vi "TLB Native Dynamic Events ver 0.12.vi"() -> ()   [LabVIEW 2018]
uses:
  Labview Training Phase 2/Enum Controls/States for Action Engine.ctl
  TLB Type Definitions/State Type Definitions, for 0.26g versions and later 2.ctl
  TLB Type Definitions/Intruction Type Definitions.ctl
  TLB Type Definitions/Encoder cluster.ctl
  Experimental VI's/Archived VI's/MOTOR CONTROL NO PID Type Def.ctl
  Underlying VI's/I2C Master VI/I2C MASTER Type Def.ctl
  TLB Type Definitions/PING CLUSTER.ctl
  <vilib>/Studica/Studica Toolkit/NavX/NavX.lvlib
  <vilib>/Studica/Studica Toolkit/Background/DIO Channel.ctl
  Underlying VI's/NavX VI/navX type def.ctl
  <vilib>/myRIO/Instrument Drivers/Utilities/Utilities.lvlib
  <vilib>/Studica/Studica Toolkit/Background/I2C Channel.ctl
  <vilib>/Studica/Studica Toolkit/NavX/TypeDefs/Flags/Z900_navX_Flags_CalibrationStatusTypeDef.ctl
  <vilib>/Studica/Studica Toolkit/NavX/TypeDefs/Flags/Z900_navX_Flags_OpStatusTypeDef.ctl
panel:
  out "Detect?":bool
  out "Status":T3 {"OP Status" items=["INITIALIZING", "SELFTEST_IN_PROGRESS", "ERROR", "IMU_AUTOCAL_IN_PROGRESS", "NORMAL"]; "Calibration Status" items=["IMU_CAL_STATE_MASK"=3, "IMU_CAL_STATE_INPROGRESS"=0, "IMU_CAL_STATE_ACCUMULATE"=1, "IMU_CAL_STATE_COMPLETE"=2]}
  out "NavX Readings":T4
  out "TASK ENABLE":bool
  out "Rising Edge":bool
  in  "Green LED":bool
  out "Task Selection":u8
  out "Object detected?":bool
  in  "Arduino Mode":T5=enum."Mode 0"
  out "Arduino Data":T6
  out "I2C Error":errorcluster
  out "Speed & distance":T7
  out "State Logic":T8=enum."Startup"
  out "elements":T9[](array[typedef])
  in  "STOP TASK":bool
  in  "OK Button":bool
  in  "STOP":bool
  out "error out":errorcluster
  out "Action Queue Items":i32
  out "State Logic Queue Items":i32
  out "Action Queues items":string[](array[string])=["Hardware reset", "Software reset", ""]
  out "Action State":string
  # "TLB FRAMEWORK STATUS"
  # "System Health Status Update"
  # "Test Programme written by Calvin Loke    Dated: 28 Aug 2019\nTest Programme revised by Dr Alex See   Dated 30 Aug 2019\n\nProgramme version:   TLB Native Dynamic Events ver 0.04b.vi"
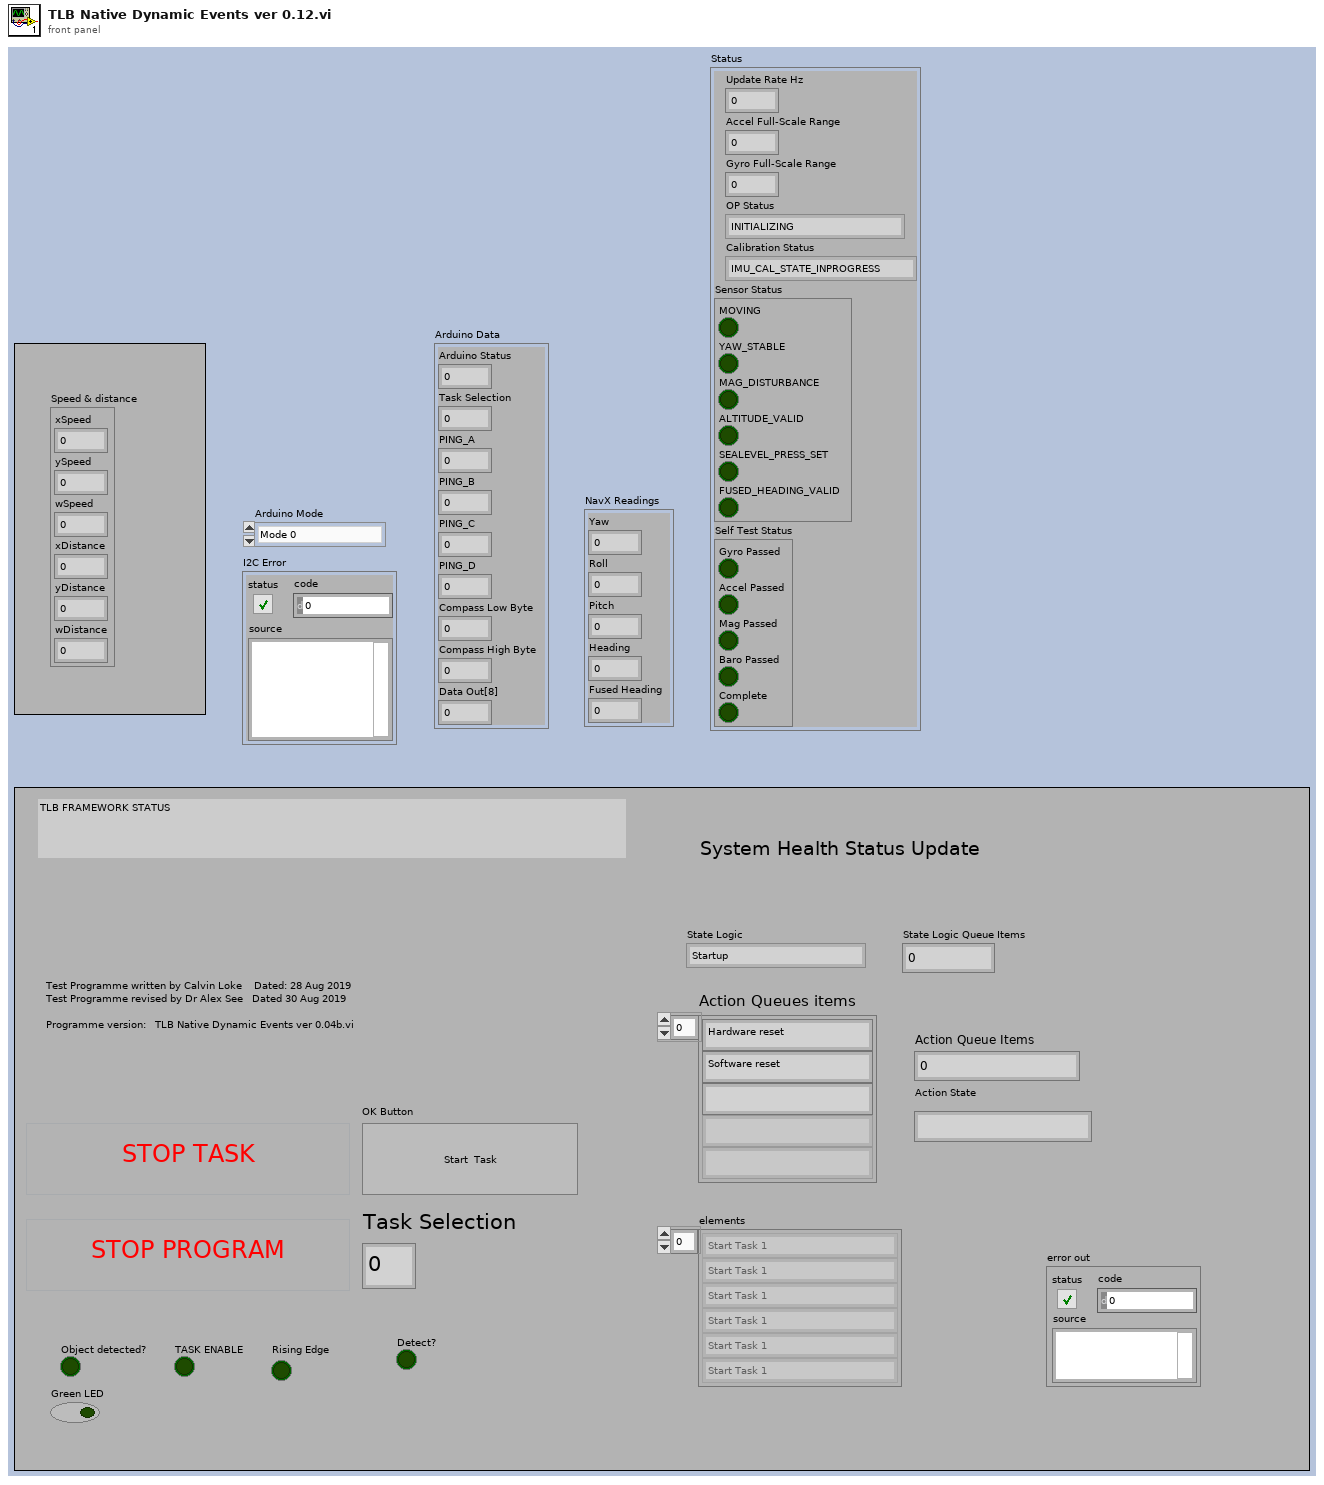
[diagram p1: front panel]
types:
  T1 = typedef "NavX.lvlib/Z900_navX_Flags_OpStatusTypeDef.ctl" = u8
  T2 = typedef "NavX.lvlib/Z900_navX_Flags_CalibrationStatusTypeDef.ctl" = u8
  T3 = cluster{"Update Rate Hz":u8, "Accel Full-Scale Range":u8, "Gyro Full-Scale Range":u16, "OP Status":T1, "Calibration Status":T2, "Sensor Status":cluster{"MOVING":bool, "YAW_STABLE":bool, "MAG_DISTURBANCE":bool, "ALTITUDE_VALID":bool, "SEALEVEL_PRESS_SET":bool, "FUSED_HEADING_VALID":bool}, "Self Test Status":cluster{"Gyro Passed":bool, "Accel Passed":bool, "Mag Passed":bool, "Baro Passed":bool, "Complete":bool}}
  T4 = cluster{"Yaw":dbl, "Roll":dbl, "Pitch":dbl, "Heading":dbl, "Fused Heading":dbl}
  T5 = typedef "I2C MASTER Type Def.ctl" = enum16{"Last State", "Mode 0", "Mode 1", "Mode 2", "Mode 3", "Mode 4", "Mode 5", "Mode 6", "Mode 7", "Mode 8", "Mode 9", "Mode 10"}
  T6 = cluster{"Arduino Status":u8, "Task Selection":u8, "PING_A":u8, "PING_B":u8, "PING_C":u8, "PING_D":u8, "Compass Low Byte":u8, "Compass High Byte":u8, "Data Out[8]":u8}
  T7 = cluster{"xSpeed":dbl, "ySpeed":dbl, "wSpeed":dbl, "xDistance":dbl, "yDistance":dbl, "wDistance":dbl}
  T8 = typedef "State Type Definitions, for 0.26g versions and later 2.ctl" = enum16{"None", "Startup", "Move to Angle", "True Stop", "Idle", "Shutdown", "Task 1A", "Task 1B", "Task 2:Raise Arm", "Task 2:Sensor Mode", "Task 2:Reverse Mode", "Task 3", "Task 4_A", "Task 4_B", "Task 4_C", "Task 4_D", "Task 5A", "Task 5B", "Task 5C", "Task 5D", "Task 5E: POSITION ARM", "Task 5F: ARM GRAB HEIGHT", "Task 5G: CLOSE CLAW", "Task 5H: RAISE ARM", "Task 6_A", "Task 6_B", "Task 7", "Task 8A: RAISE ARM", "Task 8B: MOVE TO BOX", "Task 8C: CAM BURST", "Task 8D: PROCESS IMAGE", "Task 8E: ROBOT ADJUST", "Task 8F: CAM BURST 2", "Task 8G: PROCESS IMAGE 2", "Task 8H: ARM ADJUST", "Task 8I: ARM GRAB HEIGHT", "Task 8J: CLOSE CLAW", "Task 8K: RAISE MY SWORD", "Task 9A: Raise Arm", "Task 9B: Rotate to Angle", "Task 9C: Detect Box", "Task 9D: MOVE FORWARD", "Task 9E: MOVE LEFT", "Task 9F: SCAN BOX", "Task 9G: MOVE RIGHT", "Task 9H: SCAN BOX 2", "Task 9I: ROTATE 90 CW", "Task 9J: FORWARD", "Task 9K: MOVE RIGHT", "Task 9L: SCAN BOX 3", "Task 9M: MOVE RIGHT", "Task 9N: SCAN BOX 4", "PENIS", "PENIS 2", "PENIS 3", "Task 9R: PROCESS COLOUR", "Task A1: Task 9 Open cam", "Task A2: Task 9 Move Arm", "Task A3: Task 9 Set Timer", "Task A4: Tasl 9 Capture images", "Task A5: Task 9 Close camera", "Task A6: Process Colour", "Task A7: Dispose Camera Buffer"}
  T9 = typedef "Intruction Type Definitions.ctl" = enum16{"None", "Start Task 1", "Start Task 2", "Start Task 3", "Start Task 4", "Start Task 5", "Start Task 6", "Start Task 7", "Start Task 8 - BALL", "Start Task 8 - Gel", "Start Task 8 - Pipe", "Start Task 8 - Soap", "Start Task 9", "Start Task A", "Start Task B", "Exit"}
  T10 = typedef "States for Action Engine.ctl" = enum16{"Initialize", "Write", "Read"}
  T11 = typedef "DIO Channel.ctl" = enum16{"Not Connected", "A/DIO1", "A/DIO2", "A/DIO3", "A/DIO4", "A/DIO5", "A/DIO6", "A/DIO7", "A/DIO13", "B/DIO1", "B/DIO2", "B/DIO3", "B/DIO4", "B/DIO5", "B/DIO6", "B/DIO7", "B/DIO13", "C/DIO0", "C/DIO1", "C/DIO2", "C/DIO3", "C/DIO4", "C/DIO5", "C/DIO6", "C/DIO7"}
  T12 = typedef "PING CLUSTER.ctl" = cluster{"PING_A":u8, "PING_B":u8, "PING_C":u8, "PING_D":u8}
  T13 = typedef "Encoder cluster.ctl" = cluster{"xDistance":dbl, "yDistance":dbl, "wDistance":dbl}
  T14 = typedef "I2C Channel.ctl" = enum16{"Not Connected", "A", "B"}
  T15 = typedef "navX type def.ctl" = enum16{"Get i2C reference", "Read Values", "Zero Yaw"}
  T16 = typedef "State Type Definitions.ctl" = enum16{"None", "Startup", "Move to Angle", "True Stop", "Idle", "Shutdown", "Task 1", "Task 2:Raise Arm", "Task 2:Sensor Mode", "Task 2:Reverse Mode", "Task 3", "Task 4_A", "Task 4_B", "Task 4_C", "Task 4_D", "Task 5A: ARM CAM HEIGHT", "Task 5B: MOVE TO BOX", "Task 5C: CAM BURST", "Task 5D: PROCESS IMAGE", "Task 5E: POSITION ARM", "Task 5F: ARM GRAB HEIGHT", "Task 5G: CLOSE CLAW", "Task 5H: RAISE ARM", "Task 6_A", "Task 6_B", "Task 7", "Task 8A: RAISE ARM", "Task 8B: MOVE TO BOX", "Task 8C: CAM BURST", "Task 8D: PROCESS IMAGE", "Task 8E: ROBOT ADJUST", "Task 8F: CAM BURST 2", "Task 8G: PROCESS IMAGE 2", "Task 8H: ARM ADJUST", "Task 8I: ARM GRAB HEIGHT", "Task 8J: CLOSE CLAW", "Task 8K: RAISE MY SWORD", "Task 9A: Raise Arm", "Task 9B: Rotate to Angle", "Task 9C: Detect Box", "Task 9D: MOVE FORWARD", "Task 9E: MOVE LEFT", "Task 9F: SCAN IMAGE", "Task 9G: PROCESS COLOUR", "Task 9H: MOVE RIGHT", "Task 9I: SCAN IMAGE", "Task 9J: PROCESS COLOUR", "Task 9K: ROTATE 90 CW", "Task 9L: MOVE FORWARD", "Task 9M: MOVE RIGHT", "Task 9N: SCAN IMAGE", "Task 9O: PROCESS COLOUR", "Task 9P: MOVE RIGHT", "Task 9Q: SCAN IMAGE", "Task 9R: PROCESS COLOUR"}
  T17 = typedef "State Type Definitions.ctl" = enum16{"None", "Startup", "Move to Angle", "True Stop", "Idle", "Shutdown", "Task 1", "Task 2", "Task 3", "Task 4_A", "Task 4_B", "Task 4_C", "Task 5", "Task 6", "Task 7", "Task 8", "Task 9", "Task A", "Task B"}
  T18 = typedef "MOTOR CONTROL NO PID Type Def.ctl" = enum16{"Init", "Front Back", "Left Right", "Rotate", "Stop", "Latch"}
  T19 = cluster{"DIO Channel":T11, "FPGA VI Reference Out":refnum<k20>}
  T20 = cluster{"I2C Ref Out":cluster{"I2C Channel":T14, "FPGA VI Reference Out":refnum<k20>}, "Connected":bool, "Slave Address (7-bit)":u8, "Registry":u8[]}
  T21 = cluster{"Arduino State":u8, "Rotary Switch":u8, "Ultrasonic 1":u8, "Ultrasonic 2":u8, "Ultrasonic 3":u8, "Ultrasonic 4":u8, "y Stepper Position":u8, "z Stepper Position":u8, "Data Out[8]":u8}
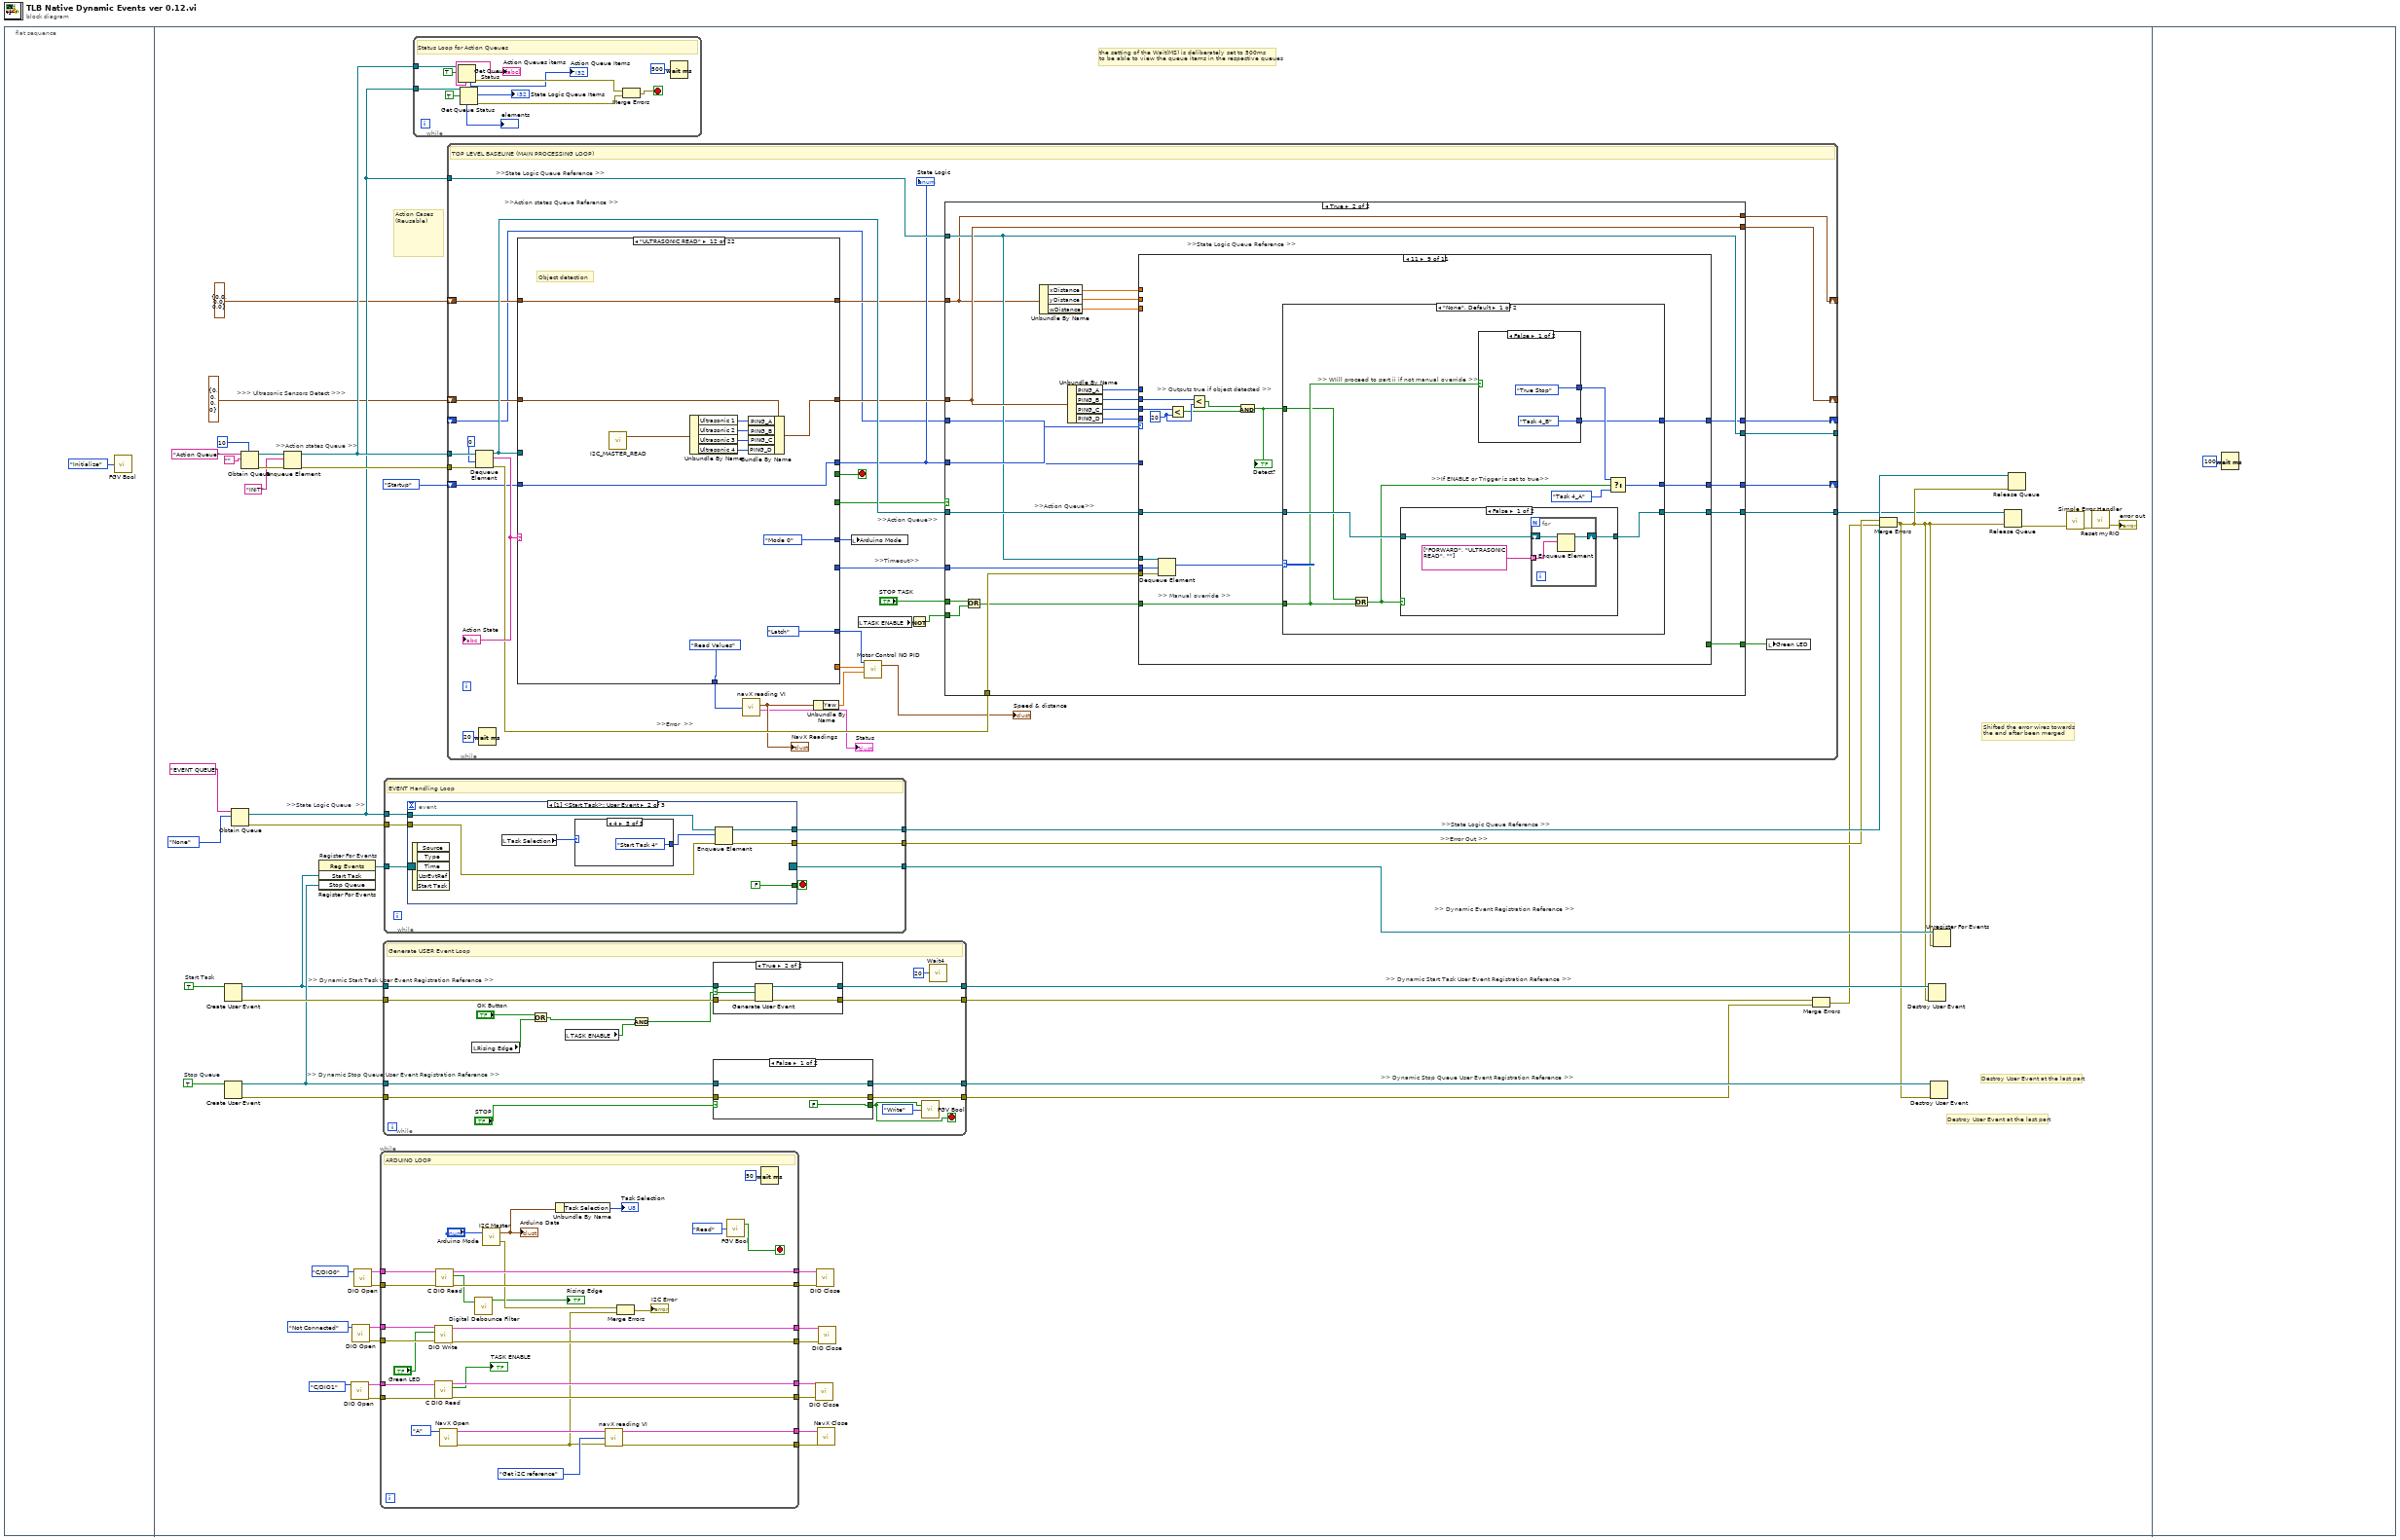
[diagram p0: block diagram]
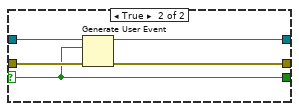
[diagram p2: hidden frame]
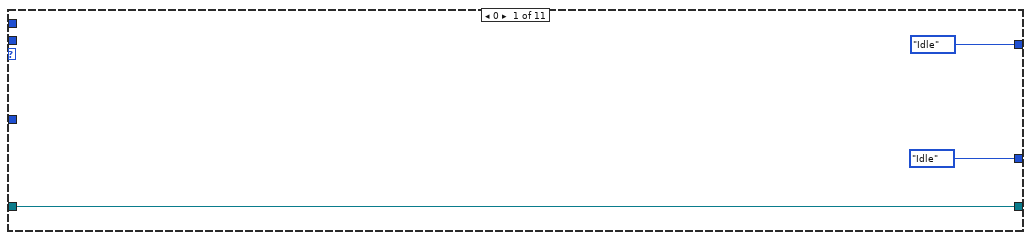
[diagram p5: hidden frame]
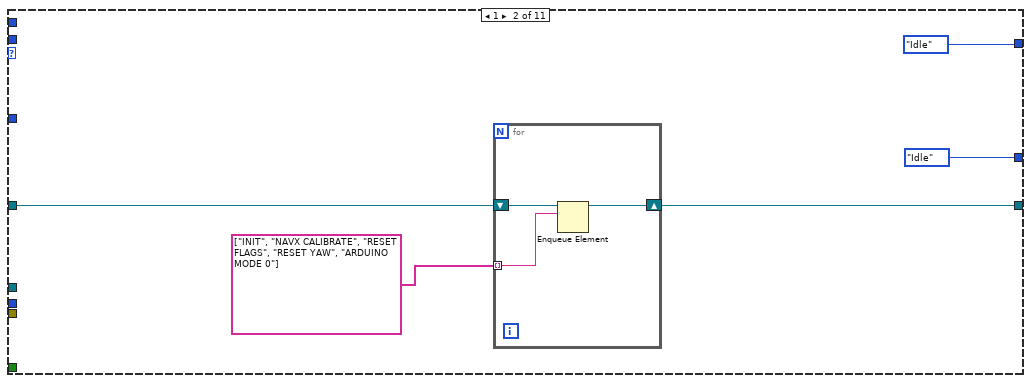
[diagram p6: hidden frame]
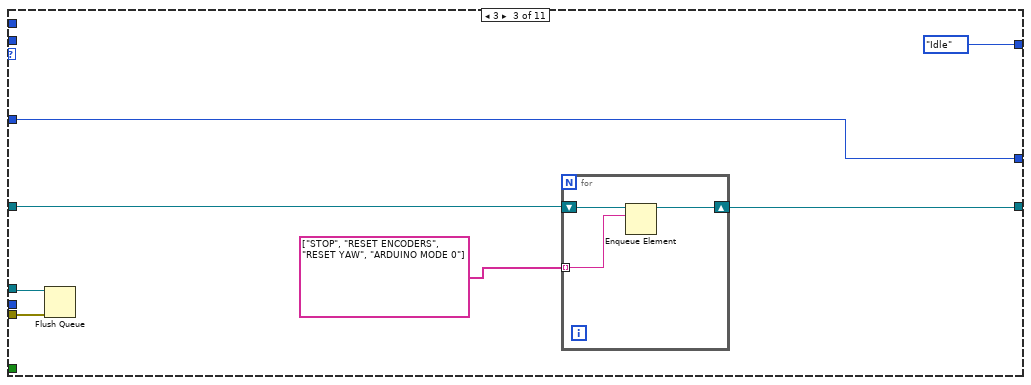
[diagram p7: hidden frame]
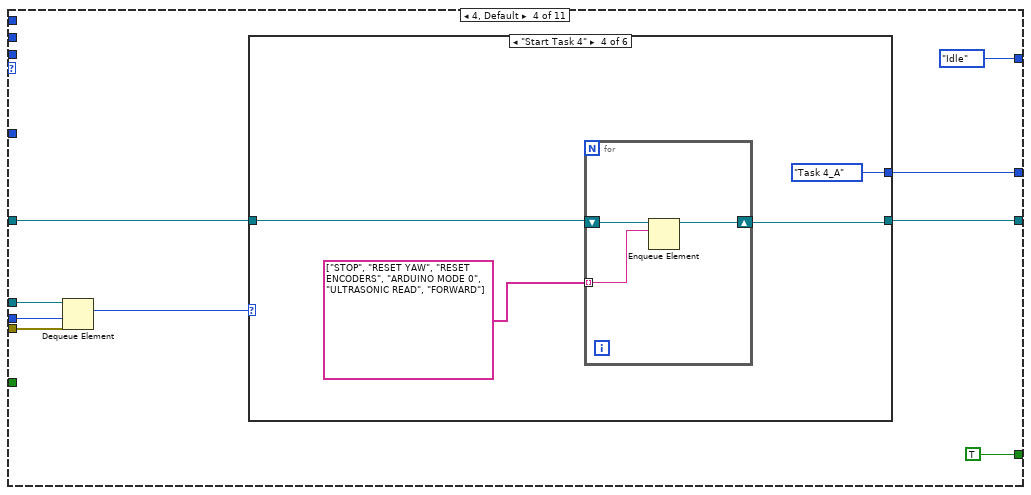
[diagram p8: hidden frame]
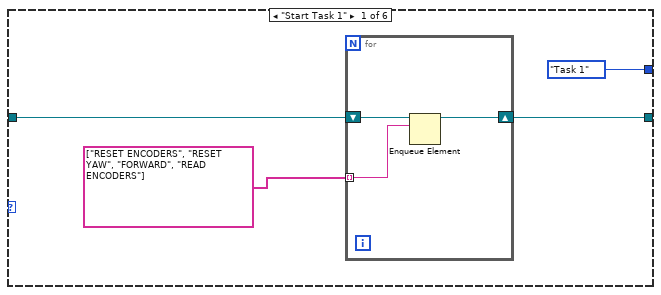
[diagram p9: hidden frame]
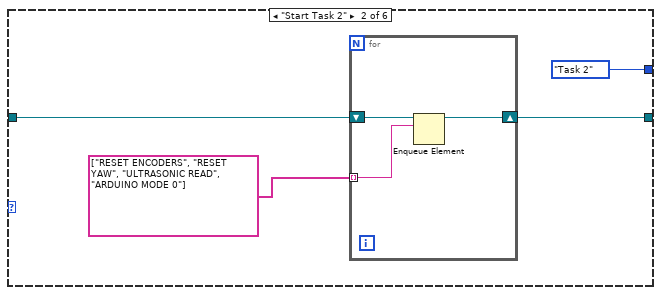
[diagram p10: hidden frame]
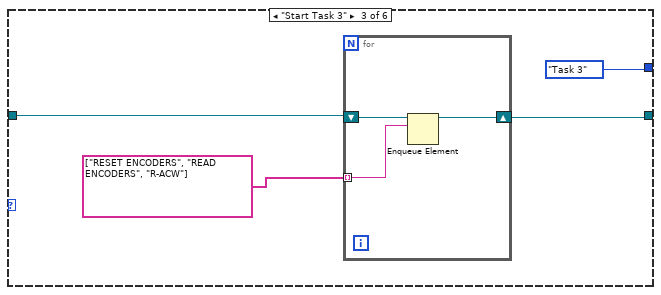
[diagram p11: hidden frame]
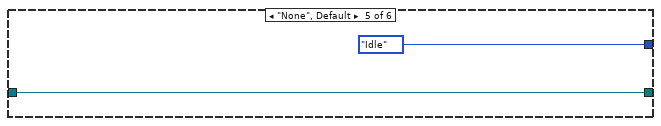
[diagram p12: hidden frame]
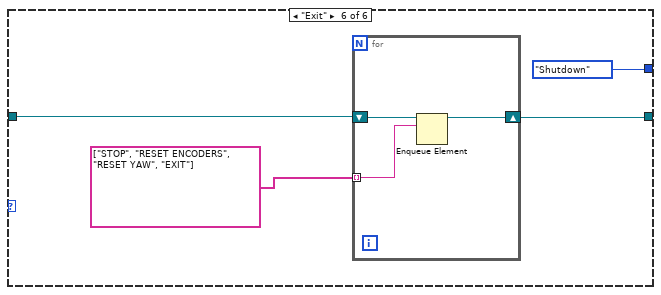
[diagram p13: hidden frame]
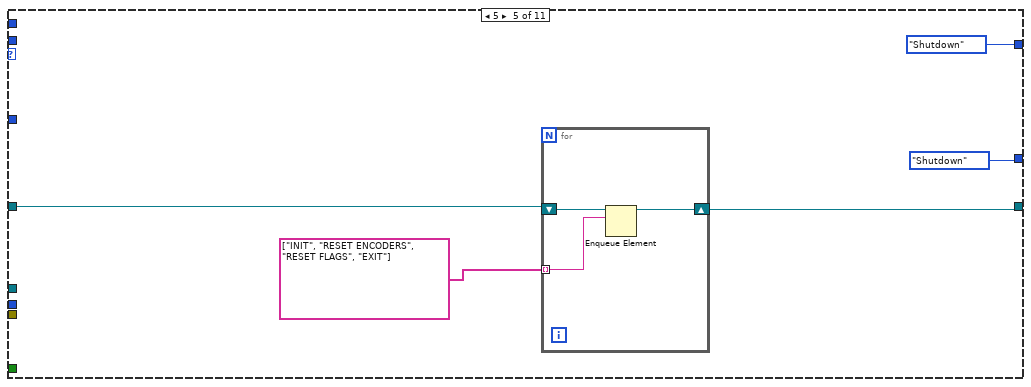
[diagram p14: hidden frame]
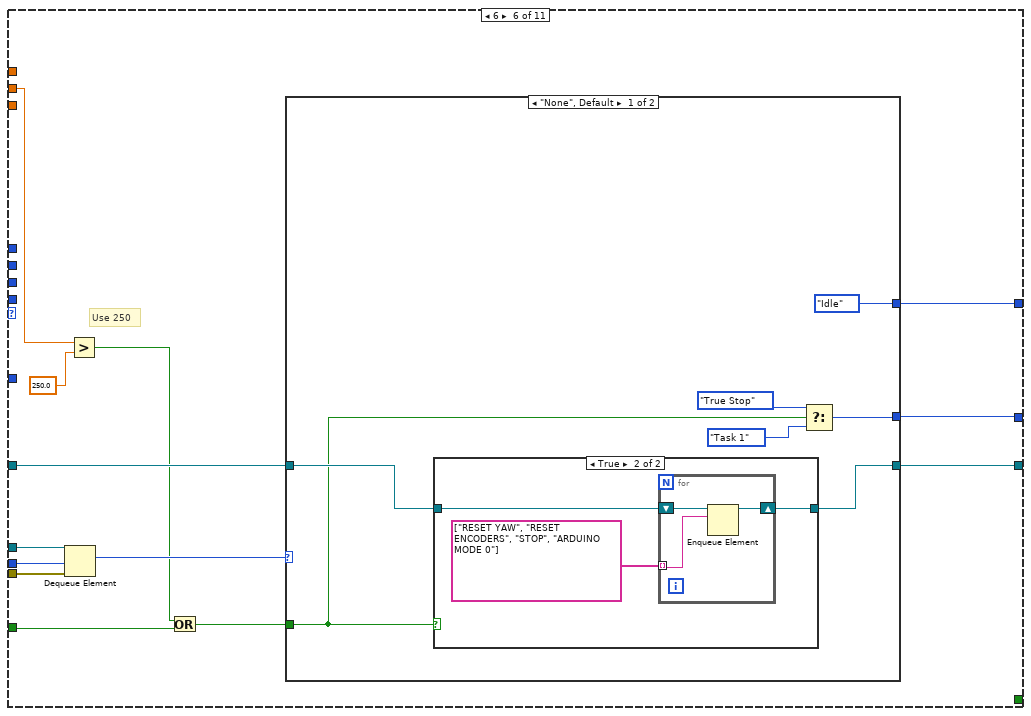
[diagram p15: hidden frame]
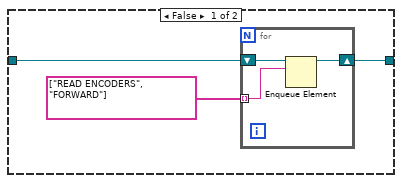
[diagram p16: hidden frame]
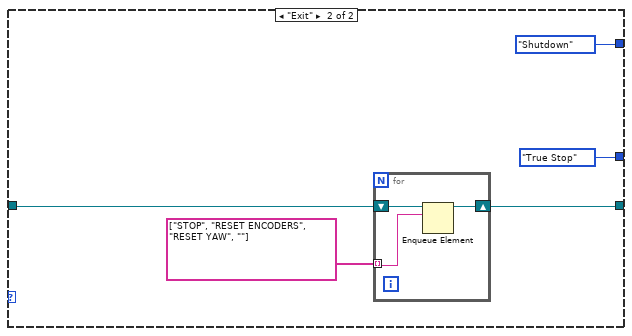
[diagram p17: hidden frame]
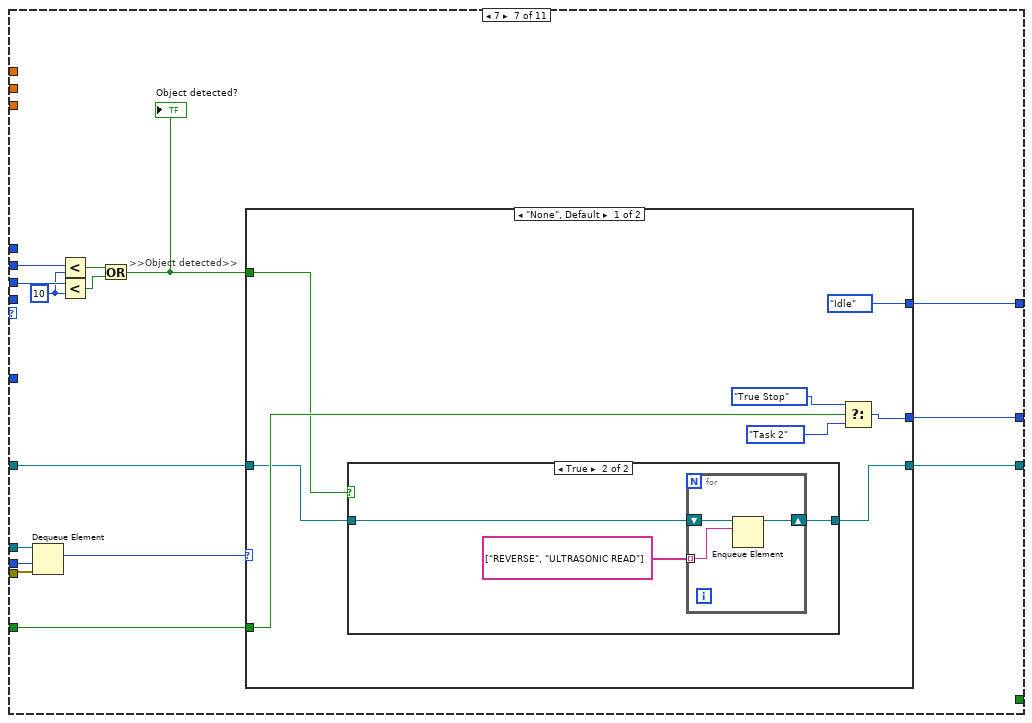
[diagram p18: hidden frame]
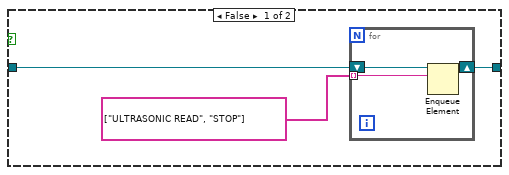
[diagram p19: hidden frame]
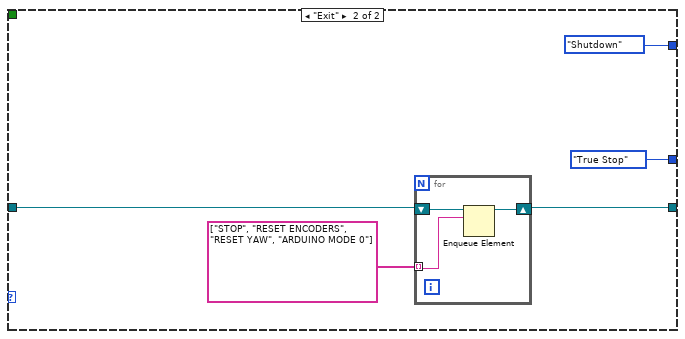
[diagram p20: hidden frame]
diagram:
  n1 = flat-sequence {
    frame #0 {
      n2 = call "FGV Bool.vi"("Init/Read/Write State"=States_for_Action_Engine."Initialize") -> ()  [unwired: 2 in, 2 out]
    }
    frame #1 {
      w53 = TRUE  # Stop Queue
      w52 = TRUE  # Start Task
      # ">>> Ultrasonic Sensors Detect >>>"
      # "the setting of the Wait(MS) is deliberately set to 500ms\nto be able to view the queue items in the respective queues"
      # "Action Cases\n(Reusable)"
      # ">>Error Out >>"
      # ">> Dynamic Stop Queue User Event Registration Reference >>"
      # ">> Dynamic Start Task User Event Registration Reference >>"
      # ">> Dynamic Stop Queue User Event Registration Reference >>"
      # ">> Dynamic Start Task User Event Registration Reference >>"
      # ">> Dynamic Event Registration Reference >>"
      # ">>Action states Queue >>"
      # ">>State Logic Queue  >>"
      # ">>State Logic Queue Reference >>"
      # "Destroy User Event at the last part"
      # "Destroy User Event at the last part"
      # "Shifted the error wires towards\nthe end after been merged"
      n3 = Create User Event(user event datatype=w52) -> (user event=w44:refnum<user-event>, error out=w49:errorcluster)  [unwired: 1 in]
      n4 = Create User Event(user event datatype=w53) -> (user event=w45:refnum<user-event>, error out=w48:errorcluster)  [unwired: 1 in]
      n5 = Obtain Queue(name (unnamed)="EVENT QUEUE", element data type=Intruction_Type_Definitions."None" ("Enum")) -> (queue out=w30:refnum<queue>, error out=w36:errorcluster)  [unwired: 3 in, 1 out]
      n6 = Obtain Queue(max queue size (-1, unlimited)=10, name (unnamed)="Action Queue", element data type="") -> (queue out=w39:refnum<queue>, error out=w35:errorcluster)  [unwired: 2 in, 1 out]
      n7 = Enqueue Element(queue=w39, element="INIT", error in (no error)=w35) -> (queue out=w31:refnum<queue>, error out=w34:errorcluster)  [unwired: 1 in, 1 out]
      n8 = register-events "Register For Events"(w44, w45) -> (reference out=w43:refnum<event-registration>)  [unwired: 2 in, 1 out]
      n9 = call <vilib>:"DIO Open.vi"("DIO Channel"=DIO_Channel."C/DIO1") -> ("error out"=w8:errorcluster, "DIO Info Out"=w9:T19)  [unwired: 9 in]
      n10 = call <vilib>:"DIO Open.vi"("DIO Channel"=DIO_Channel."Not Connected") -> ("error out"=w13:errorcluster, "DIO Info Out"=w15:T19)  [unwired: 9 in]
      n11 = call <vilib>:"DIO Open.vi"("DIO Channel"=DIO_Channel."C/DIO0") -> ("error out"=w18:errorcluster, "DIO Info Out"=w21:T19)  [unwired: 9 in]
      n12 = while {
        tunnel: w21 -> [w78]
        tunnel: [w77] -> w19
        tunnel: w18 -> [w76]
        tunnel: [w75] -> w17
        tunnel: w15 -> [w69]
        tunnel: [w68] -> w14
        tunnel: w13 -> [w67]
        tunnel: [w66] -> w12
        tunnel: [w64] -> w10
        tunnel: w9 -> [w63]
        tunnel: w8 -> [w62]
        tunnel: [w61] -> w7
        tunnel: [w58] -> w6
        tunnel: [w57] -> w5
        stop <- w82 stop-if-true
        # "ARDUINO LOOP"
        n13 = call <vilib>:"DIO Write.vi"("error in (no error)"=w67, "Input"="Green LED", "DIO Info In"=w69) -> ("error out"=w66:errorcluster, "DIO Info Out"=w68:T19)  [unwired: 7 in]
        n14 = call <vilib>:"C DIO Read.vi"("error in (no error)"=w62, "DIO Info In in"=w63) -> ("error out"=w61:errorcluster, "IN"=→"TASK ENABLE":bool, "DIO Info In out"=w64:T19)  [unwired: 7 in]
        n15 = call <vilib>:"C DIO Read.vi"("error in (no error)"=w76, "DIO Info In in"=w78) -> ("error out"=w75:errorcluster, "IN"=w72:bool, "DIO Info In out"=w77:T19)  [unwired: 7 in]
        n16 = call <vilib>:"NavX Open.vi"("I2C Channel"=I2C_Channel."A") -> ("error out"=w55:errorcluster, "NavX Info"=w59:T20)  [unwired: 9 in]
        n17 = call "Digital Debounce Filter.vi"("Boolean input"=w72) -> ("Rising Edge"=→"Rising Edge":bool)  [unwired: 1 in, 2 out]
        n18 = call "I2C Master.vi"("Arduino Mode"="Arduino Mode") -> ("I2C Error"=w74:errorcluster, "Arduino Data"=w70:T6)  [unwired: 1 in]
        "Arduino Data" <- w70
        n19 = Unbundle By Name(w70) -> ("Task Selection"=→"Task Selection":u8)
        n20 = call "navX reading VI.vi"("NavX Info In"=w59, "Mode"=navX_type_def."Get i2C reference", "error in (no error)"=w55) -> ("NavX Info Out"=w58:T20, "Error Out"=w57:errorcluster)  [unwired: 2 out]
        n21 = Merge Errors(w74, w55) -> (→"I2C Error":errorcluster)
        n22 = call "FGV Bool.vi"("Init/Read/Write State"=States_for_Action_Engine."Read") -> ("Output node"=w82:bool)  [unwired: 2 in, 1 out]
        n23 = Wait (ms)(milliseconds to wait=u32 50) -> ()  [unwired: 1 out]
      }
      n24 = while {
        tunnel: w44 -> [w112]
        tunnel: w45 -> [w111]
        tunnel: [w110] -> w51
        tunnel: [w109] -> w50
        tunnel: w49 -> [w108]
        tunnel: [w107] -> w47
        tunnel: w48 -> [w106]
        tunnel: [w105] -> w46
        stop <- w103 stop-if-true
        # "Generate USER Event Loop"
        n25 = local read "Rising Edge"() -> (w99:bool)
        n26 = Or(x="OK Button", y=w99) -> (x .or. y?=w98:bool)
        n27 = local read "TASK ENABLE"() -> (w97:bool)
        n28 = And(x=w98, y=w97) -> (x .and. y?=w96:bool)
        n29 = case shown="True" w96 {
          selector: w96 -> [_ w123]
          tunnel: w112 -> [w122 w127]
          tunnel: [w122 w126] -> w109
          tunnel: w108 -> [w121 w125]
          tunnel: [w121 w124] -> w107
          frame False {
          }
          frame True {
            n30 = Generate User Event(user event=w127, event data cluster=w123, error in=w125) -> (user event out=w126:refnum<user-event>, error out=w124:errorcluster)  [unwired: 1 in]
          }
        }
        n31 = case shown="False" "STOP" {
          selector: "STOP" -> [_ w116]
          tunnel: w111 -> [w115 w120]
          tunnel: [w115 w119] -> w110
          tunnel: w106 -> [w114 w118]
          tunnel: [w114 w117] -> w105
          tunnel: [FALSE w116] -> w103
          frame False {
          }
          frame True {
            n32 = Generate User Event(user event=w120, event data cluster=w116, error in=w118) -> (user event out=w119:refnum<user-event>, error out=w117:errorcluster)  [unwired: 1 in]
          }
        }
        n33 = call "FGV Bool.vi"("Init/Read/Write State"=States_for_Action_Engine."Write", "Input Node"=w103) -> ()  [unwired: 1 in, 2 out]
        n34 = call "Wait4"("Count(uSec)"=u32 20) -> ()  [unwired: 1 out]
      }
      n35 = while {
        tunnel: w43 -> [w685]
        tunnel: [w684] -> w42
        tunnel: w30 -> [w682]
        tunnel: [w681] -> w41
        tunnel: w36 -> [w680]
        tunnel: [w679] -> w33
        stop <- w683 stop-if-true
        # "EVENT Handling Loop"
        n36 = event shown="[1] <Start Task>: User Event" {
          selector: w685 -> [_ _ _]
          dyn-events: [_ _ _] -> w684
          timeout: _ -> [_ _ _]
          tunnel: [FALSE FALSE w709] -> w683
          tunnel: w682 -> [w690 w697 w707]
          tunnel: [w689 w696 w708] -> w681
          tunnel: w680 -> [w688 w695 w706]
          tunnel: [w687 w694 w705] -> w679
          event Timeout {
            n37 = event-data() -> ()  [unwired: 1 in, 3 out]
            n38 = Enqueue Element(queue=w690, element=Intruction_Type_Definitions."None" ("Enum"), error in (no error)=w688) -> (queue out=w689:refnum<queue>, error out=w687:errorcluster)  [unwired: 1 in, 1 out]
          }
          event User Event {
            n39 = event-data() -> ()  [unwired: 1 in, 5 out]
            n40 = local read "Task Selection"() -> (w692:u8)
            n41 = case shown="4" w692 {
              tunnel: [Intruction_Type_Definitions."None" ("Enum") Intruction_Type_Definitions."Start Task 1" ("Enum") Intruction_Type_Definitions."Start Task 2" ("Enum") Intruction_Type_Definitions."Start Task 3" ("Enum") Intruction_Type_Definitions."Start Task 4" ("Enum")] -> w693
              frame 0, Default {
              }
              frame 1 {
              }
              frame 2 {
              }
              frame 3 {
              }
              frame 4 {
              }
            }
            n42 = Enqueue Element(queue=w697, element=w693, error in (no error)=w695) -> (queue out=w696:refnum<queue>, error out=w694:errorcluster)  [unwired: 1 in, 1 out]
          }
          event User Event {
            n43 = event-data() -> ("Stop Queue"=w709:bool)  [unwired: 1 in, 4 out]
            n44 = Enqueue Element At Opposite End(queue=w707, element=Intruction_Type_Definitions."Exit" ("Enum"), error in (no error)=w706) -> (queue out=w708:refnum<queue>, error out=w705:errorcluster)  [unwired: 1 in, 1 out]
          }
        }
      }
      n45 = while {
        tunnel: w31 -> [w93]
        tunnel: w30 -> [w90]
        stop <- w87 stop-if-true
        # "Status Loop for Action Queues"
        n46 = Get Queue Status(queue=w93, return elements? (F)=TRUE) -> (error out=w89:errorcluster, # elements in queue=→"Action Queue Items":i32, elements=→"Action Queues items":string[])  [unwired: 1 in, 5 out]
        n47 = Get Queue Status(queue=w90, return elements? (F)=TRUE) -> (# pending remove=→"State Logic Queue Items":i32, error out=w88:errorcluster, elements=→"elements":T9[])  [unwired: 1 in, 5 out]
        n48 = Merge Errors(w89, w88) -> (w87:errorcluster)
        n49 = Wait (ms)(milliseconds to wait=u32 500) -> ()  [unwired: 1 out]
      }
      n50 = while {
        tunnel: w30 -> [w151]
        tunnel: w31 -> [w163]
        tunnel: w34 -> [w161]
        tunnel: [w160] -> _
        tunnel: [w159] -> w24
        shift-right: [w152] -> _
        shift-left: T12 {"PING_A"=0, "PING_B"=0, "PING_C"=0, "PING_D"=0} -> [w154]
        shift-right: [w145] -> _
        shift-left: State_Type_Definitions,_for_0.26g_versions_and_later_2."Startup" ("Enum") -> [w148]
        shift-right: [w141] -> _
        shift-left: T13 {"xDistance"=0.0, "yDistance"=0.0, "wDistance"=0.0} -> [w143]
        shift-right: [w134] -> _
        shift-left: _ -> [w133]
        stop <- w150 stop-if-true
        # ">>Error  >>"
        # ">>Action Queue>>"
        # ">>Timeout>>"
        # ">>Action states Queue Reference >>"
        # ">>State Logic Queue Reference >>"
        # "TOP LEVEL BASELINE (MAIN PROCESSING LOOP)"
        n51 = Dequeue Element(queue=w163, timeout in ms (-1)=0, error in (no error)=w161) -> (queue out=w155:refnum<queue>, element=w162:string, error out=w156:errorcluster)  [unwired: 1 out]
        "Action State" <- w162
        n52 = Wait (ms)(milliseconds to wait=u32 20) -> ()  [unwired: 1 out]
        n53 = case shown="\"ULTRASONIC READ\"" w162 {
          tunnel: [_ _ _ _ _ _ _ _ _ _ _ _ _ _ _ _ 0 w652 _ _ _ _] -> w158
          tunnel: w155 -> [_ _ _ _ _ _ _ _ _ _ _ _ _ _ _ _ _ _ _ _ _ _]
          tunnel: w154 -> [w540 w545 w552 w558 w564 w569 w576 w583 w589 w592 w604 w615 w619 w629 w633 w637 w645 w653 w658 w663 w670 w678]
          tunnel: [w540 w545 w552 w558 w564 w569 w576 w583 w589 w592 w604 w616 w619 w630 w633 w637 w645 w653 w658 w663 w669 w678] -> w153
          tunnel: [TRUE TRUE _ _ _ _ _ _ _ _ _ _ _ _ _ _ _ _ _ _ _ _] -> w150
          tunnel: w148 -> [w538 w543 w551 w557 w563 w568 w575 w582 w588 w591 w603 w614 w618 w628 w632 w636 w642 w650 w657 w662 w668 w677]
          tunnel: [_ _ _ _ _ _ _ _ _ _ _ _ _ _ _ _ _ TRUE _ _ _ _] -> w147
          tunnel: [w538 w543 w551 w557 w563 w568 w575 w582 w588 w591 w603 w614 w618 w628 w632 w636 w642 w650 w657 w662 w668 w677] -> w146
          tunnel: w143 -> [w537 w542 w550 w556 w562 w567 w574 w581 w587 w593 w602 w613 w620 w627 w634 w638 w641 w649 w659 w664 w667 w676]
          tunnel: [w537 w542 w550 w556 w562 w567 w574 w581 w587 w593 w601 w613 w620 w626 w634 w638 w641 w649 w659 w664 w667 w676] -> w142
          tunnel: [_ _ 0.4 ("Speed") -0.3 ("Speed") 0.19999999999999998 ("Speed") -0.2 ("Speed") _ 0.3 ("Speed") -0.5 ("Speed") _ _ _ _ 0.0 ("Speed") _ _ _ _ _ _ _ _] -> w140
          tunnel: [_ _ MOTOR_CONTROL_NO_PID_Type_Def."Front Back" ("Direction") _ MOTOR_CONTROL_NO_PID_Type_Def."Rotate" ("Direction") _ MOTOR_CONTROL_NO_PID_Type_Def."Stop" ("Direction") MOTOR_CONTROL_NO_PID_Type_Def."Left Right" ("Direction") MOTOR_CONTROL_NO_PID_Type_Def."Front Back" ("Direction") _ MOTOR_CONTROL_NO_PID_Type_Def."Latch" ("Direction") MOTOR_CONTROL_NO_PID_Type_Def."Latch" ("Direction") _ _ _ _ _ MOTOR_CONTROL_NO_PID_Type_Def."Latch" ("Direction") _ MOTOR_CONTROL_NO_PID_Type_Def."Init" ("Direction") _ MOTOR_CONTROL_NO_PID_Type_Def."Init" ("Direction")] -> w138
          tunnel: [I2C_MASTER_Type_Def."Last State" ("Arduino Mode") I2C_MASTER_Type_Def."Last State" ("Arduino Mode") I2C_MASTER_Type_Def."Last State" ("Arduino Mode") I2C_MASTER_Type_Def."Last State" ("Arduino Mode") I2C_MASTER_Type_Def."Last State" ("Arduino Mode") I2C_MASTER_Type_Def."Last State" ("Arduino Mode") I2C_MASTER_Type_Def."Last State" ("Arduino Mode") I2C_MASTER_Type_Def."Last State" ("Arduino Mode") I2C_MASTER_Type_Def."Last State" ("Arduino Mode") I2C_MASTER_Type_Def."Last State" ("Arduino Mode") I2C_MASTER_Type_Def."Last State" ("Arduino Mode") I2C_MASTER_Type_Def."Mode 0" ("Arduino Mode") I2C_MASTER_Type_Def."Last State" ("Arduino Mode") I2C_MASTER_Type_Def."Last State" ("Arduino Mode") I2C_MASTER_Type_Def."Mode 0" ("Arduino Mode") I2C_MASTER_Type_Def."Mode 1" ("Arduino Mode") I2C_MASTER_Type_Def."Last State" ("Arduino Mode") I2C_MASTER_Type_Def."Last State" ("Arduino Mode") I2C_MASTER_Type_Def."Last State" ("Arduino Mode") I2C_MASTER_Type_Def."Last State" ("Arduino Mode") I2C_MASTER_Type_Def."Last State" ("Arduino Mode") I2C_MASTER_Type_Def."Last State" ("Arduino Mode")] -> w137
          tunnel: [_ _ navX_type_def."Read Values" ("Mode") navX_type_def."Read Values" ("Mode") _ _ navX_type_def."Read Values" ("Mode") navX_type_def."Read Values" ("Mode") _ _ navX_type_def."Read Values" ("Mode") navX_type_def."Read Values" ("Mode") _ navX_type_def."Zero Yaw" ("Mode") _ _ navX_type_def."Zero Yaw" ("Mode") navX_type_def."Read Values" ("Mode") _ _ _ navX_type_def."Zero Yaw" ("Mode")] -> w131
          frame "Exit" {
          }
          frame "----Movement States----" {
          }
          frame "FORWARD" {
          }
          frame "LEFT" {
          }
          frame "R-ACW" {
          }
          frame "R-CW" {
          }
          frame "STOP" {
            n54 = Wait (ms)(milliseconds to wait=u32 200) -> ()  [unwired: 1 out]
          }
          frame "RIGHT" {
          }
          frame "REVERSE" {
          }
          frame "----SENSOR READING---- " {
          }
          frame "READ ENCODERS" {
            # ">>> Current encoder distance >>>"
            # ">>> Ultrasonic Sensors Detect >>>"
            n55 = local read "Speed & distance"() -> (w600:T7)
            n56 = Unbundle By Name(w600) -> ("xDistance"=w599:dbl, "yDistance"=w598:dbl, "wDistance"=w597:dbl)
            n57 = Bundle By Name(cluster=w602, "xDistance"=w599, "yDistance"=w598, "wDistance"=w597) -> (w601:T13)
          }
          frame "ULTRASONIC READ" {
            # "Object detection"
            n58 = call "I2C_MASTER_READ.vi"() -> ("Arduino Data"=w609:T21)  [unwired: 1 in, 1 out]
            n59 = Unbundle By Name(w609) -> ("Ultrasonic 1"=w608:u8, "Ultrasonic 2"=w607:u8, "Ultrasonic 3"=w606:u8, "Ultrasonic 4"=w605:u8)
            n60 = Bundle By Name(cluster=w615, "PING_A"=w608, "PING_B"=w607, "PING_C"=w606, "PING_D"=w605) -> (w616:T12)
          }
          frame "----SYSTEM MODES----" {
          }
          frame "INIT" {
            w623 = 0
            w625 = 0.0
            # ">>State Logic  >>"
            n61 = Bundle By Name(cluster=w629, "PING_A"=w623, "PING_B"=w623, "PING_C"=w623, "PING_D"=w623) -> (w630:T12)
            n62 = Bundle By Name(cluster=w627, "xDistance"=w625, "yDistance"=w625, "wDistance"=w625) -> (w626:T13)
          }
          frame "ARDUINO MODE 0" {
          }
          frame "ARDUINO MODE 1" {
          }
          frame "NAVX CALIBRATE" {
            # "Adds a 15 second delay to the startup process \nfor the NavX to calibrate"
            n63 = Wait (ms)(milliseconds to wait=u32 5000) -> ()  [unwired: 1 out]
          }
          frame "NO ACTION", Default {
            n64 = case shown="4" w650 {
              tunnel: [0 100] -> w652
              frame 1, Default {
              }
              frame 4 {
              }
            }
          }
          frame "----RESET CASES----" {
          }
          frame "RESET ENCODERS" {
          }
          frame "RESET FLAGS" {
            w666 = 0
            # "Resets any software variables\nand/or non-critical states"
            n65 = Wait (ms)(milliseconds to wait=u32 20) -> ()  [unwired: 1 out]
            n66 = Bundle By Name(cluster=w670, "PING_A"=w666, "PING_B"=w666, "PING_C"=w666, "PING_D"=w666) -> (w669:T12)
          }
          frame "RESET YAW" {
            n67 = Wait (ms)(milliseconds to wait=u32 100) -> ()  [unwired: 1 out]
          }
        }
        "State Logic" <- w146
        n68 = call "navX reading VI.vi"("Mode"=w131) -> ("NavX Readings"=w132:T4, "Status"=→"Status":T3)  [unwired: 2 in, 2 out]
        "NavX Readings" <- w132
        n69 = Unbundle By Name(w132) -> ("Yaw"=w130:dbl)
        n70 = local write "Arduino Mode"(w137) -> ()
        n71 = local read "TASK ENABLE"() -> (w136:bool)
        n72 = call "Motor Control NO PID.vi"("Yaw"=w130, "Speed"=w140, "Direction"=w138) -> ("Speed & distance"=→"Speed & distance":T7)  [unwired: 1 in, 1 out]
        n73 = Not(x=w136) -> (.not. x?=w135:bool)
        n74 = case shown="True" w147 {
          tunnel: w151 -> [w169 w186]
          tunnel: w155 -> [w165 w188]
          tunnel: [w169 w186] -> w160
          tunnel: [w165 w189] -> w159
          tunnel: w156 -> [_ w184]
          tunnel: w158 -> [_ w185]
          tunnel: w153 -> [w168 w191]
          tunnel: [w168 w191] -> w152
          tunnel: "STOP TASK" -> [_ w174]
          tunnel: w146 -> [w167 w190]
          tunnel: [w167 w187] -> w145
          tunnel: w142 -> [w166 w180]
          tunnel: [w166 w180] -> w141
          tunnel: w135 -> [_ w175]
          tunnel: [w164 w172] -> w134
          tunnel: w133 -> [w164 w171]
          tunnel: [_ w170] -> w128
          frame False {
          }
          frame True {
            # ">>Action Queue>>"
            # ">>State Logic Queue Reference >>"
            n75 = Or(x=w174, y=w175) -> (x .or. y?=w173:bool)
            n76 = Unbundle By Name(w180) -> ("xDistance"=w177:dbl, "yDistance"=w178:dbl, "wDistance"=w179:dbl)
            n77 = Unbundle By Name(w191) -> ("PING_A"=w183:u8, "PING_B"=w182:u8, "PING_C"=w181:u8, "PING_D"=w176:u8)
            n78 = case shown="11" w190 {
              tunnel: [w193 w196 w207 w215 w260 w272 w308 w354 w398 w455 w492] -> w189
              tunnel: w188 -> [w193 w199 w208 w218 w262 w273 w309 w355 w404 w448 w496]
              tunnel: [State_Type_Definitions,_for_0.26g_versions_and_later_2."Idle" ("Enum") State_Type_Definitions,_for_0.26g_versions_and_later_2."Idle" ("Enum") w203 w217 State_Type_Definitions,_for_0.26g_versions_and_later_2."Shutdown" ("Enum") w274 w311 w353 w399 w454 w493] -> w187
              tunnel: w186 -> [_ _ w206 w221 _ w279 w321 w362 w403 w452 w497]
              tunnel: w185 -> [_ _ _ w220 _ w278 w320 w361 w402 w451 w489]
              tunnel: w184 -> [_ _ w205 w216 _ w277 w319 w360 w401 w450 w488]
              tunnel: w173 -> [_ _ _ _ _ w271 w310 w357 w397 w453 w494]
              tunnel: w183 -> [_ _ _ _ _ _ _ _ _ _ _]
              tunnel: w182 -> [_ _ _ _ _ _ w317 _ w395 w443 w499]
              tunnel: w181 -> [_ _ _ _ _ _ w316 _ w396 w444 w498]
              tunnel: w179 -> [_ _ _ _ _ _ _ w359 _ _ _]
              tunnel: w178 -> [_ _ _ _ _ w270 _ _ _ _ _]
              tunnel: w177 -> [_ _ _ _ _ _ _ _ _ w439 _]
              tunnel: w176 -> [_ _ _ _ _ _ _ _ _ _ _]
              tunnel: [State_Type_Definitions,_for_0.26g_versions_and_later_2."Idle" ("Enum") State_Type_Definitions,_for_0.26g_versions_and_later_2."Idle" ("Enum") State_Type_Definitions,_for_0.26g_versions_and_later_2."Idle" ("Enum") State_Type_Definitions,_for_0.26g_versions_and_later_2."Idle" ("Enum") State_Type_Definitions,_for_0.26g_versions_and_later_2."Shutdown" ("Enum") w267 w307 w350 w390 w438 w491] -> w172
              tunnel: w171 -> [_ _ w203 _ _ _ _ _ _ _ _]
              tunnel: [_ _ _ TRUE ("Green LED") _ _ _ _ _ _ _] -> w170
              frame 0 {
              }
              frame 1 {
                n79 = for {
                  shift-right: [w202] -> w196
                  shift-left: w199 -> [w201]
                  tunnel: string[] ["INIT", "NAVX CALIBRATE", "RESET FLAGS", "RESET YAW", "ARDUINO MODE 0"] -> [w200] mode=indexing
                  n80 = Enqueue Element(queue=w201, element=w200) -> (queue out=w202:refnum<queue>)  [unwired: 2 in, 2 out]
                }
              }
              frame 3 {
                n81 = Flush Queue(queue=w206, error in (no error)=w205) -> ()  [unwired: 3 out]
                n82 = for {
                  shift-right: [w212] -> w207
                  shift-left: w208 -> [w211]
                  tunnel: string[] ["STOP", "RESET ENCODERS", "RESET YAW", "ARDUINO MODE 0"] -> [w210] mode=indexing
                  n83 = Enqueue Element(queue=w211, element=w210) -> (queue out=w212:refnum<queue>)  [unwired: 2 in, 2 out]
                }
              }
              frame 4, Default {
                n84 = Dequeue Element(queue=w221, timeout in ms (-1)=w220, error in (no error)=w216) -> (element=w219:T9)  [unwired: 3 out]
                n85 = case shown="\"Start Task 4\"" w219 {
                  tunnel: [w223 w230 w237 w244 w251 w253] -> w215
                  tunnel: w218 -> [w224 w231 w238 w245 w251 w254]
                  tunnel: [State_Type_Definitions."Task 1" ("Enum") State_Type_Definitions."Task 2" ("Enum") State_Type_Definitions,_for_0.26g_versions_and_later_2."Task 3" ("Enum") State_Type_Definitions,_for_0.26g_versions_and_later_2."Task 4_A" ("Enum") State_Type_Definitions,_for_0.26g_versions_and_later_2."Idle" ("Enum") State_Type_Definitions,_for_0.26g_versions_and_later_2."Shutdown" ("Enum")] -> w217
                  frame "Start Task 1" {
                    n86 = for {
                      shift-right: [w228] -> w223
                      shift-left: w224 -> [w227]
                      tunnel: string[] ["RESET ENCODERS", "RESET YAW", "FORWARD", "READ ENCODERS"] -> [w226] mode=indexing
                      n87 = Enqueue Element(queue=w227, element=w226) -> (queue out=w228:refnum<queue>)  [unwired: 2 in, 2 out]
                    }
                  }
                  frame "Start Task 2" {
                    n88 = for {
                      shift-right: [w235] -> w230
                      shift-left: w231 -> [w234]
                      tunnel: string[] ["RESET ENCODERS", "RESET YAW", "ULTRASONIC READ", "ARDUINO MODE 0"] -> [w233] mode=indexing
                      n89 = Enqueue Element(queue=w234, element=w233) -> (queue out=w235:refnum<queue>)  [unwired: 2 in, 2 out]
                    }
                  }
                  frame "Start Task 3" {
                    n90 = for {
                      shift-right: [w242] -> w237
                      shift-left: w238 -> [w241]
                      tunnel: string[] ["RESET ENCODERS", "READ ENCODERS", "R-ACW"] -> [w240] mode=indexing
                      n91 = Enqueue Element(queue=w241, element=w240) -> (queue out=w242:refnum<queue>)  [unwired: 2 in, 2 out]
                    }
                  }
                  frame "Start Task 4" {
                    n92 = for {
                      shift-right: [w249] -> w244
                      shift-left: w245 -> [w248]
                      tunnel: string[] ["STOP", "RESET YAW", "RESET ENCODERS", "ARDUINO MODE 0", "ULTRASONIC READ", "FORWARD"] -> [w247] mode=indexing
                      n93 = Enqueue Element(queue=w248, element=w247) -> (queue out=w249:refnum<queue>)  [unwired: 2 in, 2 out]
                    }
                  }
                  frame "None", Default {
                  }
                  frame "Exit" {
                    n94 = for {
                      shift-right: [w258] -> w253
                      shift-left: w254 -> [w257]
                      tunnel: string[] ["STOP", "RESET ENCODERS", "RESET YAW", "EXIT"] -> [w256] mode=indexing
                      n95 = Enqueue Element(queue=w257, element=w256) -> (queue out=w258:refnum<queue>)  [unwired: 2 in, 2 out]
                    }
                  }
                }
              }
              frame 5 {
                n96 = for {
                  shift-right: [w266] -> w260
                  shift-left: w262 -> [w265]
                  tunnel: string[] ["INIT", "RESET ENCODERS", "RESET FLAGS", "EXIT"] -> [w264] mode=indexing
                  n97 = Enqueue Element(queue=w265, element=w264) -> (queue out=w266:refnum<queue>)  [unwired: 2 in, 2 out]
                }
              }
              frame 6 {
                # "Use 250"
                n98 = Dequeue Element(queue=w279, timeout in ms (-1)=w278, error in (no error)=w277) -> (element=w276:T9)  [unwired: 3 out]
                n99 = Greater?(x=w270, y=250.0) -> (0:w268:bool)
                n100 = Or(x=w268, y=w271) -> (x .or. y?=w275:bool)
                n101 = case shown="\"None\", Default" w276 {
                  tunnel: w275 -> [w282 _]
                  tunnel: [w286 State_Type_Definitions,_for_0.26g_versions_and_later_2."True Stop" ("Enum")] -> w274
                  tunnel: w273 -> [w283 w301]
                  tunnel: [w281 w300] -> w272
                  tunnel: [State_Type_Definitions,_for_0.26g_versions_and_later_2."Idle" ("Enum") State_Type_Definitions,_for_0.26g_versions_and_later_2."Shutdown" ("Enum")] -> w267
                  frame "None", Default {
                    n102 = case shown="True" w282 {
                      tunnel: w283 -> [w289 w295]
                      tunnel: [w288 w293] -> w281
                      frame False {
                        n103 = for {
                          shift-right: [w291] -> w288
                          shift-left: w289 -> [w292]
                          tunnel: string[] ["READ ENCODERS", "FORWARD"] ("element") -> [w290] mode=indexing
                          n104 = Enqueue Element(queue=w292, element=w290) -> (queue out=w291:refnum<queue>)  [unwired: 2 in, 2 out]
                        }
                      }
                      frame True {
                        n105 = for {
                          shift-right: [w297] -> w293
                          shift-left: w295 -> [w298]
                          tunnel: string[] ["RESET YAW", "RESET ENCODERS", "STOP", "ARDUINO MODE 0"] -> [w296] mode=indexing
                          n106 = Enqueue Element(queue=w298, element=w296) -> (queue out=w297:refnum<queue>)  [unwired: 2 in, 2 out]
                        }
                      }
                    }
                    n107 = Select(t=State_Type_Definitions,_for_0.26g_versions_and_later_2."True Stop" ("Enum"), s=w282, f=State_Type_Definitions."Task 1" ("Enum")) -> (s? t:f=w286:u16)
                  }
                  frame "Exit" {
                    n108 = for {
                      shift-right: [w305] -> w300
                      shift-left: w301 -> [w306]
                      tunnel: string[] ["STOP", "RESET ENCODERS", "RESET YAW", ""] -> [w304] mode=indexing
                      n109 = Enqueue Element(queue=w306, element=w304) -> (queue out=w305:refnum<queue>)  [unwired: 2 in, 2 out]
                    }
                  }
                }
              }
              frame 7 {
                w315 = u16 10 ("y")
                # ">>Object detected>>"
                n110 = Dequeue Element(queue=w321, timeout in ms (-1)=w320, error in (no error)=w319) -> (element=w318:T9)  [unwired: 3 out]
                n111 = Less?(x=w317, y=w315) -> (x < y?=w314:bool)
                n112 = Less?(x=w316, y=w315) -> (x < y?=w313:bool)
                n113 = Or(x=w314, y=w313) -> (x .or. y?=w312:bool)
                "Object detected?" <- w312
                n114 = case shown="\"None\", Default" w318 {
                  tunnel: w312 -> [w325 _]
                  tunnel: [w327 State_Type_Definitions,_for_0.26g_versions_and_later_2."True Stop" ("Enum")] -> w311
                  tunnel: w310 -> [w326 _]
                  tunnel: w309 -> [w324 w344]
                  tunnel: [w323 w345] -> w308
                  tunnel: [State_Type_Definitions,_for_0.26g_versions_and_later_2."Idle" ("Enum") State_Type_Definitions,_for_0.26g_versions_and_later_2."Shutdown" ("Enum")] -> w307
                  frame "None", Default {
                    n115 = case shown="True" w325 {
                      tunnel: w324 -> [w331 w338]
                      tunnel: [w332 w337] -> w323
                      frame False {
                        n116 = for {
                          tunnel: string[] ["ULTRASONIC READ", "STOP"] ("element") -> [w333] mode=indexing
                          shift-right: [w335] -> w332
                          shift-left: w331 -> [w334]
                          n117 = Enqueue Element(queue=w334, element=w333) -> (queue out=w335:refnum<queue>)  [unwired: 2 in, 2 out]
                        }
                      }
                      frame True {
                        n118 = for {
                          shift-right: [w340] -> w337
                          shift-left: w338 -> [w341]
                          tunnel: string[] ["REVERSE", "ULTRASONIC READ"] -> [w339] mode=indexing
                          n119 = Enqueue Element(queue=w341, element=w339) -> (queue out=w340:refnum<queue>)  [unwired: 2 in, 2 out]
                        }
                      }
                    }
                    n120 = Select(t=State_Type_Definitions,_for_0.26g_versions_and_later_2."True Stop" ("Enum"), s=w326, f=State_Type_Definitions."Task 2" ("Enum")) -> (s? t:f=w327:u16)
                  }
                  frame "Exit" {
                    n121 = for {
                      shift-right: [w348] -> w345
                      shift-left: w344 -> [w349]
                      tunnel: string[] ["STOP", "RESET ENCODERS", "RESET YAW", "ARDUINO MODE 0"] -> [w347] mode=indexing
                      n122 = Enqueue Element(queue=w349, element=w347) -> (queue out=w348:refnum<queue>)  [unwired: 2 in, 2 out]
                    }
                  }
                }
              }
              frame 10 {
                n123 = Dequeue Element(queue=w362, timeout in ms (-1)=w361, error in (no error)=w360) -> (element=w351:T9)  [unwired: 3 out]
                n124 = Greater?(x=w359, y=150.0) -> (0:w356:bool)
                n125 = Or(x=w356, y=w357) -> (x .or. y?=w352:bool)
                n126 = case shown="\"Exit\"" w351 {
                  tunnel: w352 -> [w365 _]
                  tunnel: [w369 State_Type_Definitions,_for_0.26g_versions_and_later_2."True Stop" ("Enum")] -> w353
                  tunnel: w355 -> [w366 w385]
                  tunnel: [w364 w384] -> w354
                  tunnel: [State_Type_Definitions,_for_0.26g_versions_and_later_2."Idle" ("Enum") State_Type_Definitions,_for_0.26g_versions_and_later_2."Shutdown" ("Enum")] -> w350
                  frame "None", Default {
                    n127 = case shown="False" w365 {
                      tunnel: w366 -> [w372 w378]
                      tunnel: [w371 w376] -> w364
                      frame False {
                        n128 = for {
                          shift-right: [w374] -> w371
                          shift-left: w372 -> [w375]
                          tunnel: string[] ["READ ENCODERS", "R-ACW"] ("element") -> [w373] mode=indexing
                          n129 = Enqueue Element(queue=w375, element=w373) -> (queue out=w374:refnum<queue>)  [unwired: 2 in, 2 out]
                        }
                      }
                      frame True {
                        n130 = for {
                          shift-right: [w380] -> w376
                          shift-left: w378 -> [w381]
                          tunnel: string[] ["RESET YAW", "RESET ENCODERS", "STOP", "ARDUINO MODE 0"] -> [w379] mode=indexing
                          n131 = Enqueue Element(queue=w381, element=w379) -> (queue out=w380:refnum<queue>)  [unwired: 2 in, 2 out]
                        }
                      }
                    }
                    n132 = Select(t=State_Type_Definitions,_for_0.26g_versions_and_later_2."True Stop" ("Enum"), s=w365, f=State_Type_Definitions,_for_0.26g_versions_and_later_2."Task 3" ("Enum")) -> (s? t:f=w369:T8)
                  }
                  frame "Exit" {
                    n133 = for {
                      shift-right: [w388] -> w384
                      shift-left: w385 -> [w389]
                      tunnel: string[] ["STOP", "RESET ENCODERS", "RESET YAW", ""] -> [w387] mode=indexing
                      n134 = Enqueue Element(queue=w389, element=w387) -> (queue out=w388:refnum<queue>)  [unwired: 2 in, 2 out]
                    }
                  }
                }
              }
              frame 11 {
                w394 = 20
                # ">> Outputs true if object detected >>"
                # ">> Manual override >>"
                n135 = Dequeue Element(queue=w403, timeout in ms (-1)=w402, error in (no error)=w401) -> (element=w400:T9)  [unwired: 3 out]
                n136 = Less?(x=w396, y=w394) -> (x < y?=w392:bool)
                n137 = Less?(x=w395, y=w394) -> (x < y?=w393:bool)
                n138 = And(x=w393, y=w392) -> (x .and. y?=w391:bool)
                "Detect?" <- w391
                n139 = case shown="\"None\", Default" w400 {
                  tunnel: [w413 State_Type_Definitions,_for_0.26g_versions_and_later_2."True Stop" ("Enum")] -> w399
                  tunnel: [w411 w432] -> w398
                  tunnel: w404 -> [w410 _]
                  tunnel: w397 -> [w408 _]
                  tunnel: w391 -> [w406 _]
                  tunnel: [w405 State_Type_Definitions,_for_0.26g_versions_and_later_2."Shutdown" ("Enum")] -> w390
                  frame "None", Default {
                    # ">> WIill proceed to part ii if not manual override >>"
                    # ">>If ENABLE or Trigger is set to true>>"
                    n140 = Or(x=w406, y=w408) -> (x .or. y?=w407:bool)
                    n141 = case shown="False" w407 {
                      tunnel: [w420 w425] -> w411
                      tunnel: w410 -> [w418 w424]
                      frame False {
                        n142 = for {
                          shift-right: [w422] -> w420
                          shift-left: w418 -> [w423]
                          tunnel: string[] ["FORWARD", "ULTRASONIC READ", ""] ("element") -> [w421] mode=indexing
                          n143 = Enqueue Element(queue=w423, element=w421) -> (queue out=w422:refnum<queue>)  [unwired: 2 in, 2 out]
                        }
                      }
                      frame True {
                        n144 = for {
                          shift-right: [w428] -> w425
                          shift-left: w424 -> [w429]
                          tunnel: string[] ["STOP", "RESET ENCODERS", "RESET YAW", "ARDUINO MODE 0"] -> [w427] mode=indexing
                          n145 = Enqueue Element(queue=w429, element=w427) -> (queue out=w428:refnum<queue>)  [unwired: 2 in, 2 out]
                        }
                      }
                    }
                    n146 = case shown="False" w408 {
                      tunnel: [State_Type_Definitions,_for_0.26g_versions_and_later_2."True Stop" ("Enum") State_Type_Definitions,_for_0.26g_versions_and_later_2."True Stop" ("Enum")] -> w409
                      tunnel: [State_Type_Definitions,_for_0.26g_versions_and_later_2."Task 4_B" ("Enum") State_Type_Definitions,_for_0.26g_versions_and_later_2."Idle" ("Enum")] -> w405
                      frame False {
                      }
                      frame True {
                      }
                    }
                    n147 = Select(t=w409, s=w407, f=State_Type_Definitions,_for_0.26g_versions_and_later_2."Task 4_A" ("Enum")) -> (s? t:f=w413:T8)
                  }
                  frame "Exit" {
                    n148 = for {
                      shift-right: [w435] -> w432
                      shift-left: _ -> [w436]
                      tunnel: string[] ["STOP", "RESET ENCODERS", "RESET YAW", ""] -> [w434] mode=indexing
                      n149 = Enqueue Element(queue=w436, element=w434) -> (queue out=w435:refnum<queue>)  [unwired: 2 in, 2 out]
                    }
                  }
                }
              }
              frame 12 {
                w447 = 20
                # ">> Outputs true if 150 mm has been moved >>"
                # ">> Outputs true if sensor not obstructed>>"
                # ">> Manual override >>"
                n150 = Dequeue Element(queue=w452, timeout in ms (-1)=w451, error in (no error)=w450) -> (element=w449:T9)  [unwired: 3 out]
                n151 = Greater?(x=w444, y=w447) -> (0:w445:bool)
                n152 = Greater?(x=w443, y=w447) -> (0:w446:bool)
                n153 = Greater Or Equal?(x=w439, y=80.0) -> (x >= y?=w441:bool)
                n154 = And(x=w446, y=w445) -> (x .and. y?=w440:bool)
                n155 = And(x=w441, y=w440) -> (x .and. y?=w437:bool)
                n156 = case shown="\"None\", Default" w449 {
                  tunnel: [w464 State_Type_Definitions,_for_0.26g_versions_and_later_2."True Stop" ("Enum")] -> w454
                  tunnel: [w462 w483] -> w455
                  tunnel: w448 -> [w461 _]
                  tunnel: w453 -> [w459 _]
                  tunnel: w437 -> [w457 _]
                  tunnel: [w456 State_Type_Definitions,_for_0.26g_versions_and_later_2."Shutdown" ("Enum")] -> w438
                  frame "None", Default {
                    # ">> WIill proceed to part ii if not manual override >>"
                    # ">>If ENABLE or Trigger is set to true>>"
                    n157 = Or(x=w457, y=w459) -> (x .or. y?=w458:bool)
                    n158 = case shown="False" w458 {
                      tunnel: [w471 w476] -> w462
                      tunnel: w461 -> [w469 w475]
                      frame False {
                        n159 = for {
                          shift-right: [w473] -> w471
                          shift-left: w469 -> [w474]
                          tunnel: string[] ["RIGHT", "ULTRASONIC READ", "READ ENCODERS"] ("element") -> [w472] mode=indexing
                          n160 = Enqueue Element(queue=w474, element=w472) -> (queue out=w473:refnum<queue>)  [unwired: 2 in, 2 out]
                        }
                      }
                      frame True {
                        n161 = for {
                          shift-right: [w479] -> w476
                          shift-left: w475 -> [w480]
                          tunnel: string[] ["STOP", "RESET ENCODERS", "RESET YAW", "ARDUINO MODE 0"] -> [w478] mode=indexing
                          n162 = Enqueue Element(queue=w480, element=w478) -> (queue out=w479:refnum<queue>)  [unwired: 2 in, 2 out]
                        }
                      }
                    }
                    n163 = case shown="False" w459 {
                      tunnel: [State_Type_Definitions,_for_0.26g_versions_and_later_2."True Stop" ("Enum") State_Type_Definitions,_for_0.26g_versions_and_later_2."True Stop" ("Enum")] -> w460
                      tunnel: [State_Type_Definitions,_for_0.26g_versions_and_later_2."Task 4_C" ("Enum") State_Type_Definitions,_for_0.26g_versions_and_later_2."Idle" ("Enum")] -> w456
                      frame False {
                      }
                      frame True {
                      }
                    }
                    n164 = Select(t=w460, s=w458, f=State_Type_Definitions,_for_0.26g_versions_and_later_2."Task 4_B" ("Enum")) -> (s? t:f=w464:T8)
                  }
                  frame "Exit" {
                    n165 = for {
                      shift-right: [w486] -> w483
                      shift-left: _ -> [w487]
                      tunnel: string[] ["STOP", "RESET ENCODERS", "RESET YAW", ""] -> [w485] mode=indexing
                      n166 = Enqueue Element(queue=w487, element=w485) -> (queue out=w486:refnum<queue>)  [unwired: 2 in, 2 out]
                    }
                  }
                }
              }
              frame 13 {
                w502 = 30
                # ">> Outputs true if object detected >>"
                # ">> Manual override >>"
                n167 = Dequeue Element(queue=w497, timeout in ms (-1)=w489, error in (no error)=w488) -> (element=w490:T9)  [unwired: 3 out]
                n168 = Less?(x=w498, y=w502) -> (x < y?=w500:bool)
                n169 = Less?(x=w499, y=w502) -> (x < y?=w501:bool)
                n170 = And(x=w501, y=w500) -> (x .and. y?=w495:bool)
                n171 = case shown="\"None\", Default" w490 {
                  tunnel: [w511 State_Type_Definitions,_for_0.26g_versions_and_later_2."True Stop" ("Enum")] -> w493
                  tunnel: [w509 w531] -> w492
                  tunnel: w496 -> [w508 w528]
                  tunnel: w494 -> [w506 _]
                  tunnel: w495 -> [w504 _]
                  tunnel: [w503 State_Type_Definitions,_for_0.26g_versions_and_later_2."Shutdown" ("Enum")] -> w491
                  frame "None", Default {
                    # ">> WIill proceed to part ii if not manual override >>"
                    # ">>If ENABLE or Trigger is set to true>>"
                    n172 = Or(x=w504, y=w506) -> (x .or. y?=w505:bool)
                    n173 = case shown="False" w505 {
                      tunnel: [w518 w523] -> w509
                      tunnel: w508 -> [w516 w522]
                      frame False {
                        n174 = for {
                          shift-right: [w520] -> w518
                          shift-left: w516 -> [w521]
                          tunnel: string[] ["FORWARD", "ULTRASONIC READ", ""] ("element") -> [w519] mode=indexing
                          n175 = Enqueue Element(queue=w521, element=w519) -> (queue out=w520:refnum<queue>)  [unwired: 2 in, 2 out]
                        }
                      }
                      frame True {
                        n176 = for {
                          shift-right: [w526] -> w523
                          shift-left: w522 -> [w527]
                          tunnel: string[] ["STOP", "RESET ENCODERS", "RESET YAW", "ARDUINO MODE 0"] -> [w525] mode=indexing
                          n177 = Enqueue Element(queue=w527, element=w525) -> (queue out=w526:refnum<queue>)  [unwired: 2 in, 2 out]
                        }
                      }
                    }
                    n178 = case shown="True" w506 {
                      tunnel: [State_Type_Definitions,_for_0.26g_versions_and_later_2."True Stop" ("Enum") State_Type_Definitions,_for_0.26g_versions_and_later_2."True Stop" ("Enum")] -> w507
                      tunnel: [State_Type_Definitions,_for_0.26g_versions_and_later_2."Idle" ("Enum") State_Type_Definitions,_for_0.26g_versions_and_later_2."Idle" ("Enum")] -> w503
                      frame False {
                      }
                      frame True {
                      }
                    }
                    n179 = Select(t=w507, s=w505, f=State_Type_Definitions,_for_0.26g_versions_and_later_2."Task 4_C" ("Enum")) -> (s? t:f=w511:T8)
                  }
                  frame "Exit" {
                    n180 = for {
                      shift-right: [w534] -> w531
                      shift-left: w528 -> [w535]
                      tunnel: string[] ["STOP", "RESET ENCODERS", "RESET YAW", ""] -> [w533] mode=indexing
                      n181 = Enqueue Element(queue=w535, element=w533) -> (queue out=w534:refnum<queue>)  [unwired: 2 in, 2 out]
                    }
                  }
                }
              }
            }
          }
        }
        n182 = local write "Green LED"(w128) -> ()
      }
      n183 = call <vilib>:"DIO Close.vi"("error in (no error)"=w7, "DIO Info In"=w10) -> ()  [unwired: 9 in, 1 out]
      n184 = call <vilib>:"DIO Close.vi"("error in (no error)"=w17, "DIO Info In"=w19) -> ()  [unwired: 9 in, 1 out]
      n185 = call <vilib>:"NavX Close.vi"("error in (no error)"=w5, "NavX Info In"=w6) -> ()  [unwired: 9 in, 1 out]
      n186 = call <vilib>:"DIO Close.vi"("error in (no error)"=w12, "DIO Info In"=w14) -> ()  [unwired: 9 in, 1 out]
      n187 = Merge Errors "Merge Errors"(w47, w46) -> (w29:errorcluster)
      n188 = Merge Errors(w33, w29) -> (w28:errorcluster)
      n189 = Destroy User Event(user event=w50, error in=w28) -> ()  [unwired: 1 out]
      n190 = Destroy User Event(user event=w51, error in=w28) -> ()  [unwired: 1 out]
      n191 = Unregister For Events(event registration refnum=w42, error in=w28) -> ()  [unwired: 1 out]
      n192 = Release Queue(queue=w24, error in (no error)=w28) -> (error out=w4:errorcluster)  [unwired: 1 in, 2 out]
      n193 = Release Queue(queue=w41, error in (no error)=w28) -> ()  [unwired: 1 in, 3 out]
      n194 = call <vilib>:"Simple Error Handler.vi"("error in (no error)"=w4) -> ("error out"=w3:errorcluster)  [unwired: 4 in, 4 out]
      n195 = call <vilib>:"Reset myRIO.vi"("error in (no error)"=w3) -> ("error out"=→"error out":errorcluster)  [unwired: 10 in]
    }
    frame #2 {
      n196 = Wait (ms)(milliseconds to wait=u32 100) -> ()  [unwired: 1 out]
    }
  }
